vi "TestInsertIntoPanel_OK.vi"(8 "error in (no error)":errorcluster, 11 "TestCase in":refnum<class "TestProtectedSubpanel.lvclass">) -> (0 "error out":errorcluster, 3 "TestCase out":refnum<class "TestProtectedSubpanel.lvclass">)   [LabVIEW 2015, in "TestProtectedSubpanel.lvclass"]
uses:
  TestProtectedSubpanel.lvclass
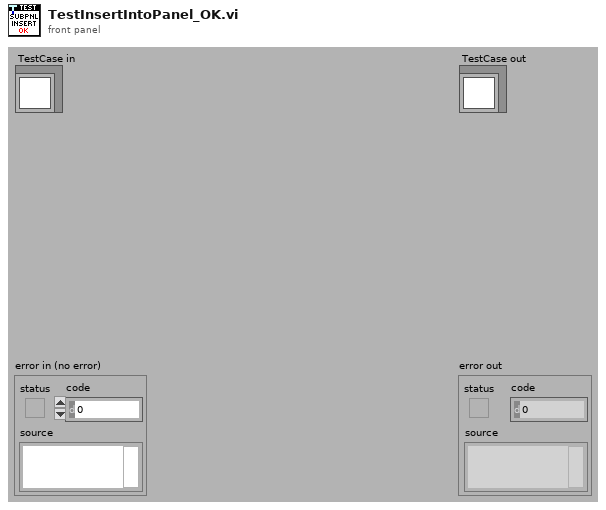
[diagram p1: front panel]
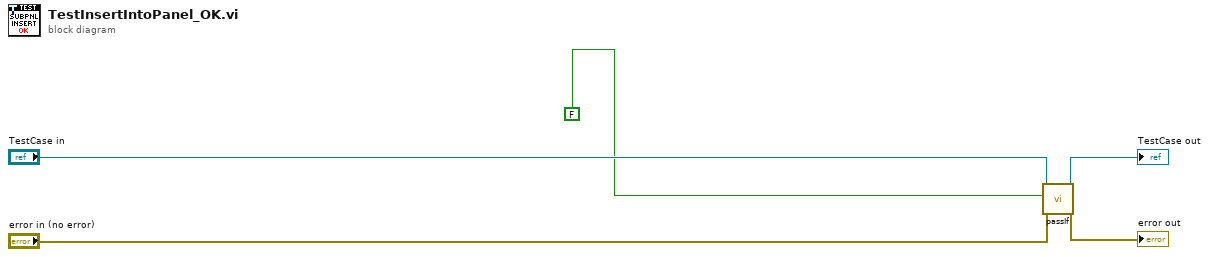
[diagram p0: block diagram]
diagram:
  n1 = call-dynamic "passIf.vi"("error in (no error)"="error in (no error)", "pass"=FALSE, "TestCase in"="TestCase in") -> ("error out"=→"error out":errorcluster, "TestCase out"=→"TestCase out":refnum<class "TestProtectedSubpanel.lvclass">)  [unwired: 7 in]
